vi "End SEQUENCE handler.vi"(7 "main seq?":bool, 11 "input sequences":string[](array[string])) -> (3 "output sequences":string[](array[string]))   [LabVIEW 2020]
panel:
  out "logical OR":bool
  out "Array":bool[](array[boolean])
  # "sub seq"
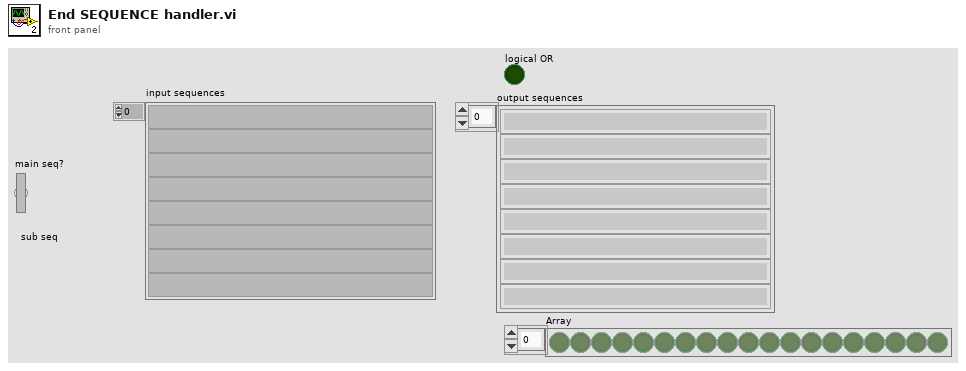
[diagram p1: front panel]
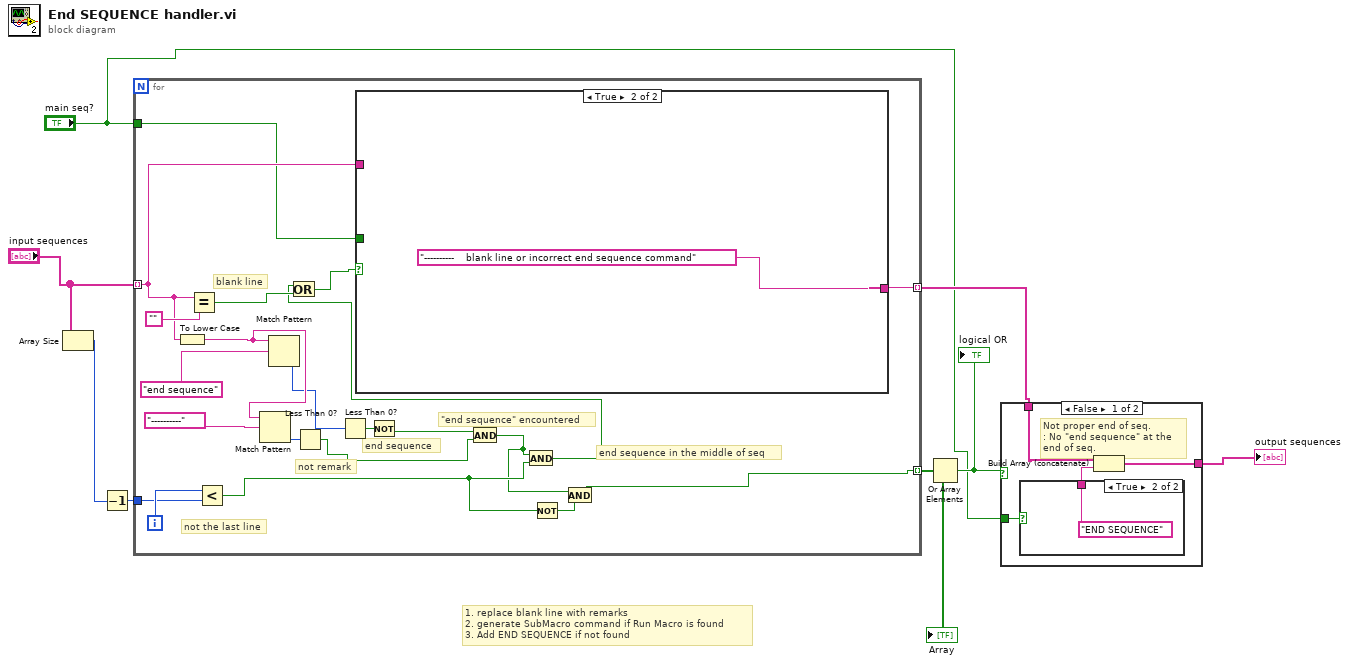
[diagram p0: block diagram]
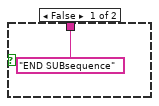
[diagram p2: hidden frame]
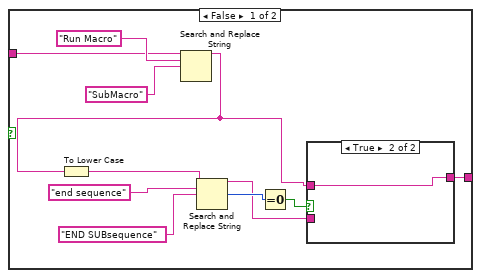
[diagram p5: hidden frame]
diagram:
  # "1. replace blank line with remarks\n2. generate SubMacro command if Run Macro is found\n3. Add END SEQUENCE if not found"
  n1 = Array Size(array="input sequences") -> (size(s)=w6:i32)
  n2 = Decrement(x=w6) -> (x-1=w5:i32)
  n3 = for {
    tunnel: "input sequences" -> [w27] mode=indexing
    tunnel: [w29] -> w3 mode=indexing
    tunnel: [w10] -> w8 mode=indexing
    tunnel: "main seq?" -> [w18]
    tunnel: w5 -> [w16]
    i -> [w17]
    # "end sequence in the middle of seq"
    # "blank line"
    # "\"end sequence\" encountered"
    # "not the last line"
    # "end sequence"
    # "not remark"
    n4 = To Lower Case(string=w27) -> (all lower case string=w25:string)
    n5 = Equal?(x=w27, y="") -> (x = y?=w15:bool)
    n6 = Less?(x=w17, y=w16) -> (x < y?=w13:bool)
    n7 = Match Pattern(string=w25, regular expression="----------") -> (offset past match=w22:i32)  [unwired: 1 in, 3 out]
    n8 = Match Pattern(string=w25, regular expression="end sequence" ("search string")) -> (offset past match=w23:i32)  [unwired: 1 in, 3 out]
    n9 = Less Than 0?(x=w22) -> (x < 0?=w19:bool)
    n10 = Less Than 0?(x=w23) -> (x < 0?=w21:bool)
    n11 = Not(x=w21) -> (.not. x?=w20:bool)
    n12 = And(x=w20, y=w19) -> (x .and. y?=w12:bool)
    n13 = And(x=w12, y=w13) -> (x .and. y?=w11:bool)
    n14 = Or(x=w11, y=w15) -> (x .or. y?=w14:bool)
    n15 = case shown="True" w14 {
      tunnel: [w32 "----------    blank line or incorrect end sequence command" ("result string")] -> w29
      tunnel: w27 -> [w31 _]
      tunnel: w18 -> [w30 _]
      frame False {
        n16 = case shown="True" w30 {
          tunnel: [w38 w46] -> w32
          tunnel: w31 -> [w33 w46]
          frame False {
            n17 = Search and Replace String(input string=w33, search string="Run Macro", replace string="SubMacro" ("replace string (\"\")")) -> (result string=w34:string)  [unwired: 5 in, 3 out]
            n18 = To Lower Case(string=w34) -> (all lower case string=w43:string)
            n19 = Search and Replace String(input string=w43, search string="end sequence", replace string="END SUBsequence" ("replace string (\"\")")) -> (result string=w37:string, number of replacements=w40:i32)  [unwired: 5 in, 2 out]
            n20 = Equal To 0?(x=w40) -> (x = 0?=w39:bool)
            n21 = case shown="True" w39 {
              tunnel: w34 -> [_ w45]
              tunnel: [w44 w45] -> w38
              tunnel: w37 -> [w44 _]
              frame False {
              }
              frame True {
              }
            }
          }
          frame True {
          }
        }
      }
      frame True {
      }
    }
    n22 = Not(x=w13) -> (.not. x?=w9:bool)
    n23 = And(x=w12, y=w9) -> (x .and. y?=w10:bool)
  }
  "Array" <- w8
  n24 = Or Array Elements(Boolean array=w8) -> (logical OR=w4:bool)
  "logical OR" <- w4
  n25 = case shown="False" w4 {
    tunnel: w3 -> [w51 w54]
    tunnel: [w49 w54] -> w1
    tunnel: "main seq?" -> [w48 _]
    frame False {
      # "Not proper end of seq.\n: No \"end sequence\" at the\nend of seq."
      n26 = case shown="True" w48 {
        tunnel: ["END SUBsequence" ("replace string (\"\")") "END SEQUENCE" ("replace string (\"\")")] -> w50
        frame False {
        }
        frame True {
        }
      }
      n27 = Build Array (concatenate)(w51, w50) -> (w49:string[])
    }
    frame True {
    }
  }
  "output sequences" <- w1
